vi "TimerStart.vi"(0 "error in (no error)":errorcluster) -> (4 "error out":errorcluster, 15 "StartTime":dbl format="%_19f")   [LabVIEW 2016, in "AssertTimer.lvlib"]
uses:
  AssertTimer.lvlib
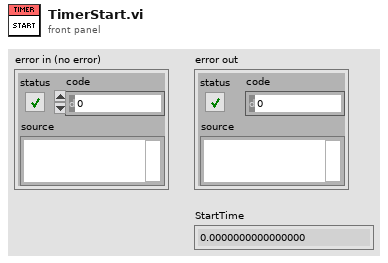
[diagram p1: front panel]
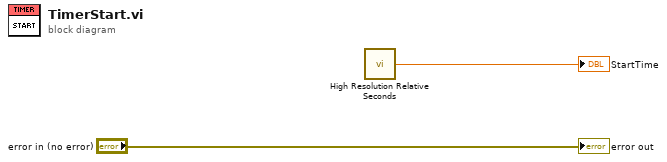
[diagram p0: block diagram]
diagram:
  n1 = call <vilib>:"High Resolution Relative Seconds.vi"() -> ("relative seconds"=→"StartTime":dbl)
  "error out" <- "error in (no error)"
